vi "From Serial Form.vi"(6 "Serial Version":T1, 10 "Deserializer in":refnum<class "Deserializer.lvclass">=refnum, 11 "AlicatCommBank in":refnum<class "AlicatCommBank.lvclass">=refnum) -> (0 "error out":errorcluster, 2 "Deserializer out":refnum<class "Deserializer.lvclass">, 3 "AlicatCommBank out":refnum<class "AlicatCommBank.lvclass">)   [LabVIEW 2014]
uses:
  Alicat.lvclass
  <userlib>/Serialization/Serializable/Remove Boolean.vi
  <userlib>/Serialization/Serialization Common/Serial Version.ctl
  <userlib>/Serialization/Deserializer/Deserializer.lvclass
  AlicatCommBank.lvclass
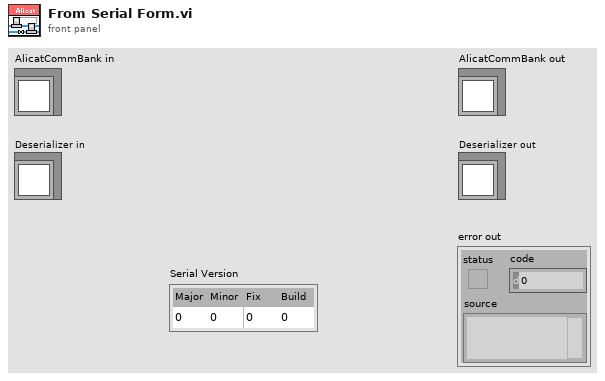
[diagram p1: front panel]
types:
  T1 = typedef "Serialization Common.lvlib/Serial Version.ctl" = cluster{"Major":u16, "Minor":u16, "Fix":u16, "Build":u16}
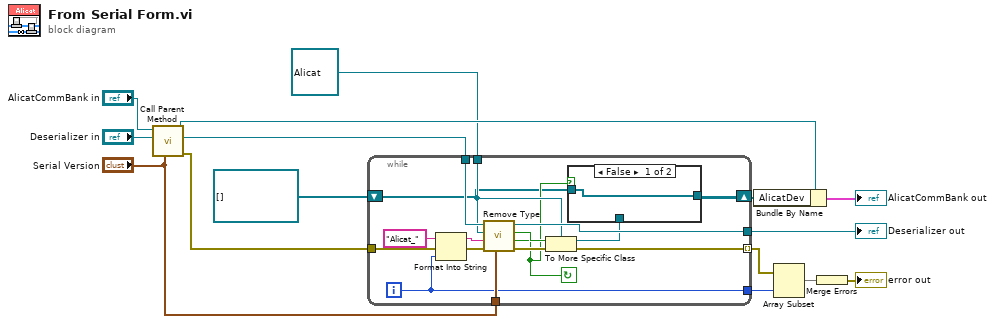
[diagram p0: block diagram]
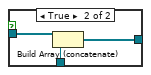
[diagram p2: hidden frame]
diagram:
  n1 = call-parent "Call Parent Method"("Serial Version"="Serial Version", "Deserializer in"="Deserializer in", "Serial IO in"="AlicatCommBank in") -> ("error out"=w8:errorcluster, "Deserializer out"=w12:refnum<class "Deserializer.lvclass">, "Serial IO out"=w13:refnum<class "AlicatCommBank.lvclass">)  [unwired: 6 in]
  n2 = while {
    tunnel: w12 -> [w29]
    tunnel: refnum<class "Alicat.lvclass"> refnum ("Alicat.lvclass") -> [w26]
    tunnel: [w28] -> w10
    tunnel: "Serial Version" -> [w22]
    shift-right: [w18] -> w9
    shift-left: refnum<class "Alicat.lvclass">[] [] -> [w19]
    tunnel: w8 -> [w24]
    tunnel: [w17] -> w4 mode=indexing
    tunnel: [w16] -> w3
    i -> [w16]
    stop <- w21 continue-if-true
    n3 = Format Into String(initial string="Alicat_", error in=w24, w16) -> (resulting string=w30:string, error out=w23:errorcluster)  [unwired: 1 in]
    n4 = call-poly <userlib>:"Remove Type.vi"(6:w22, "error in (no error)"=w23, "Name"=w30, "Default Value"=w26, "Deserializer in"=w29) -> ("error out"=w25:errorcluster, "Found?"=w21:bool, "Boolean"=w27:bool, "Deserializer out"=w28:refnum<class "Deserializer.lvclass">)  [unwired: 3 in]
    n5 = To More Specific Class(target class=w26, reference=w27, error in=w25) -> (specific class reference=w20:refnum<class "Alicat.lvclass">, error out=w17:errorcluster)
    n6 = case shown="False" w21 {
      tunnel: w20 -> [_ w35]
      tunnel: w19 -> [w32 w34]
      tunnel: [w32 w33] -> w18
      frame False {
      }
      frame True {
        n7 = Build Array (concatenate)(w34, w35) -> (w33:refnum<class "Alicat.lvclass">[])
      }
    }
  }
  "Deserializer out" <- w10
  n8 = Bundle By Name(cluster=w13, "AlicatDev"=w9) -> (→"AlicatCommBank out":cluster{})
  n9 = Array Subset(array=w4, length=w3) -> (w2:errorcluster[])  [unwired: 1 in]
  n10 = Merge Errors(w2) -> (→"error out":errorcluster)
